vi "PSRR_PMIC.vi"() -> ()   [LabVIEW 2024]
panel:
  in  "MeasGraphs":enum32{"PSRR", "Hidden Controls"}(tab)
  out "Status":string
  out "PSRR vs Frequency":T1(graph)
  in  "Scope resource name":string
  in  "Fgen resource name":string
  in  "Load resource name":string
  in  "Source resource name":string caption="RESOURCE NAME"
  in  "MeasConfigurations":T2(tab)
  in  "Load sense":string="Remote" caption="LOAD SENSE"
  in  "Source sense":string="Remote" caption="SOURCE SENSE"
  in  "Nominal output voltage":dbl=3.3 caption="NOMINAL OUTPUT VOLTAGE" format="%#_6pV"
  in  "DUT setup time":dbl=1.0 caption="DUT SETUP TIME" format="%#_6ps"
  in  "Measurement settings":string="Measurement settings"
  in  "Source configuration":string="Source configuration"
  in  "Load configuration":string="Load configuration"
  in  "Load voltage limit":dbl=5.0 caption="VOLTAGE LIMIT" format="%#_6pV"
  in  "Load current level":dbl=0.05 caption="CURRENT LEVEL" format="%#_6pA"
  in  "Load resource name":refnum<k15> caption="RESOURCE NAME"
  in  "Source current limit":dbl=0.5 caption="CURRENT LIMIT" format="%#_6pA"
  in  "Source voltage level":dbl=20.0 caption="VOLTAGE LEVEL" format="%#_6pV"
  in  "Source resource name":refnum<k15> caption="RESOURCE NAME"
  in  "Scope vout range":dbl=0.05 caption="VOUT RANGE"
  in  "Scope input impedance":dbl=1000000.0 caption="INPUT IMPEDANCE" format="%#_6pOhm"
  in  "Scope number of cycles":i32=8 caption="NUMBER OF CYCLES"
  in  "Scope samples per cycle":i32=100000 caption="SAMPLES PER CYCLE"
  in  "Scope probe attenuation Vout":dbl=1.0 caption="VOUT PROBE ATTENUATION"
  in  "Scope output channel":string caption="OUTPUT CHANNEL NAME"
  in  "Scope maximum sample rate":dbl=100000000.0 caption="MAX SAMPLE RATE"
  in  "Scope minimum sample rate":dbl=100.0 caption="MIN SAMPLE RATE"
  in  "FGEN sweep type":string(combo)="Logarithmic" caption="SWEEP TYPE"
  in  "FGEN points or points per decade":i32=10 caption="PTS/PTS PER DECADE"
  in  "FGEN stop frequency":dbl=10000000.0 caption="STOP FREQUENCY" format="%#_6pHz"
  in  "FGEN start frequency":dbl=100.0 caption="START FREQUENCY" format="%#_6pHz"
  in  "FGEN load impedance":dbl=10000.0 caption="LOAD IMPEDANCE" format="%#_6pOhm"
  in  "Fgen configuration":string="Fgen configuration"
  in  "FGEN pk-pk amplitude":dbl=1.0 caption="PK-PK AMPLITUDE" format="%#_6pV"
  in  "FGEN channel name":string="0" caption="CHANNEL NAME"
  in  "FGEN resource name":refnum<k15> caption="RESOURCE NAME"
  in  "Scope probe attenuation Vin":dbl=1.0 caption="VIN PROBE ATTENUATION"
  in  "Scope configuration":string="Scope configuration"
  in  "Scope input channel":string caption="INPUT CHANNEL NAME"
  in  "Scope resource name":refnum<k15> caption="RESOURCE NAME"
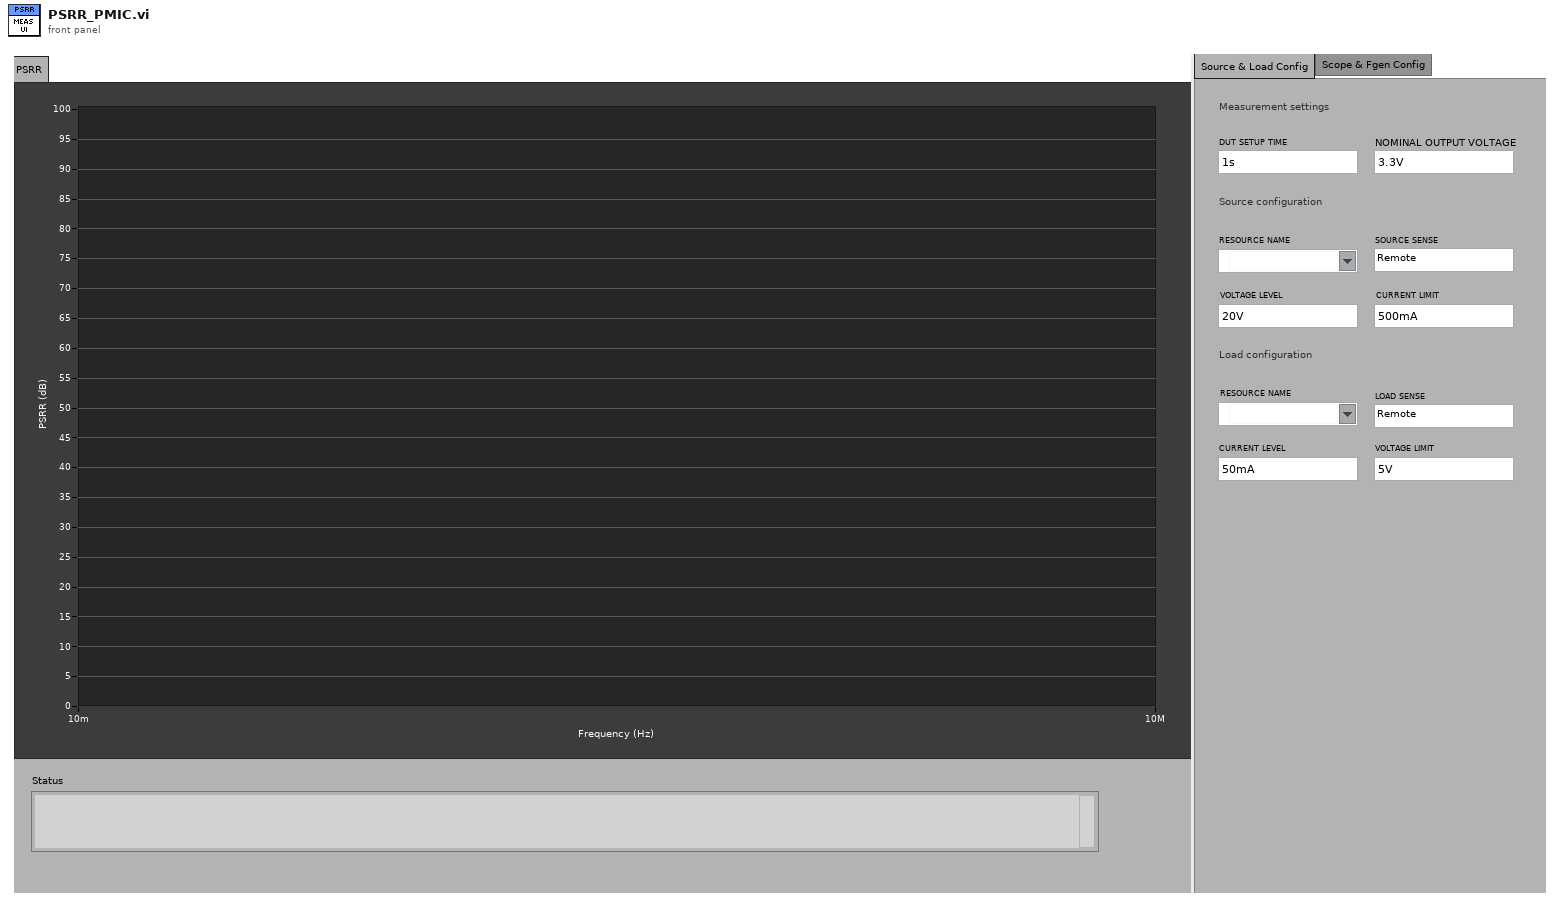
[diagram p1: front panel]
types:
  T1 = cluster{"Source voltages":dbl[], "Load voltages":dbl[]}
  T2 = enum32{"Source & Load Config", "Scope & Fgen Config"}
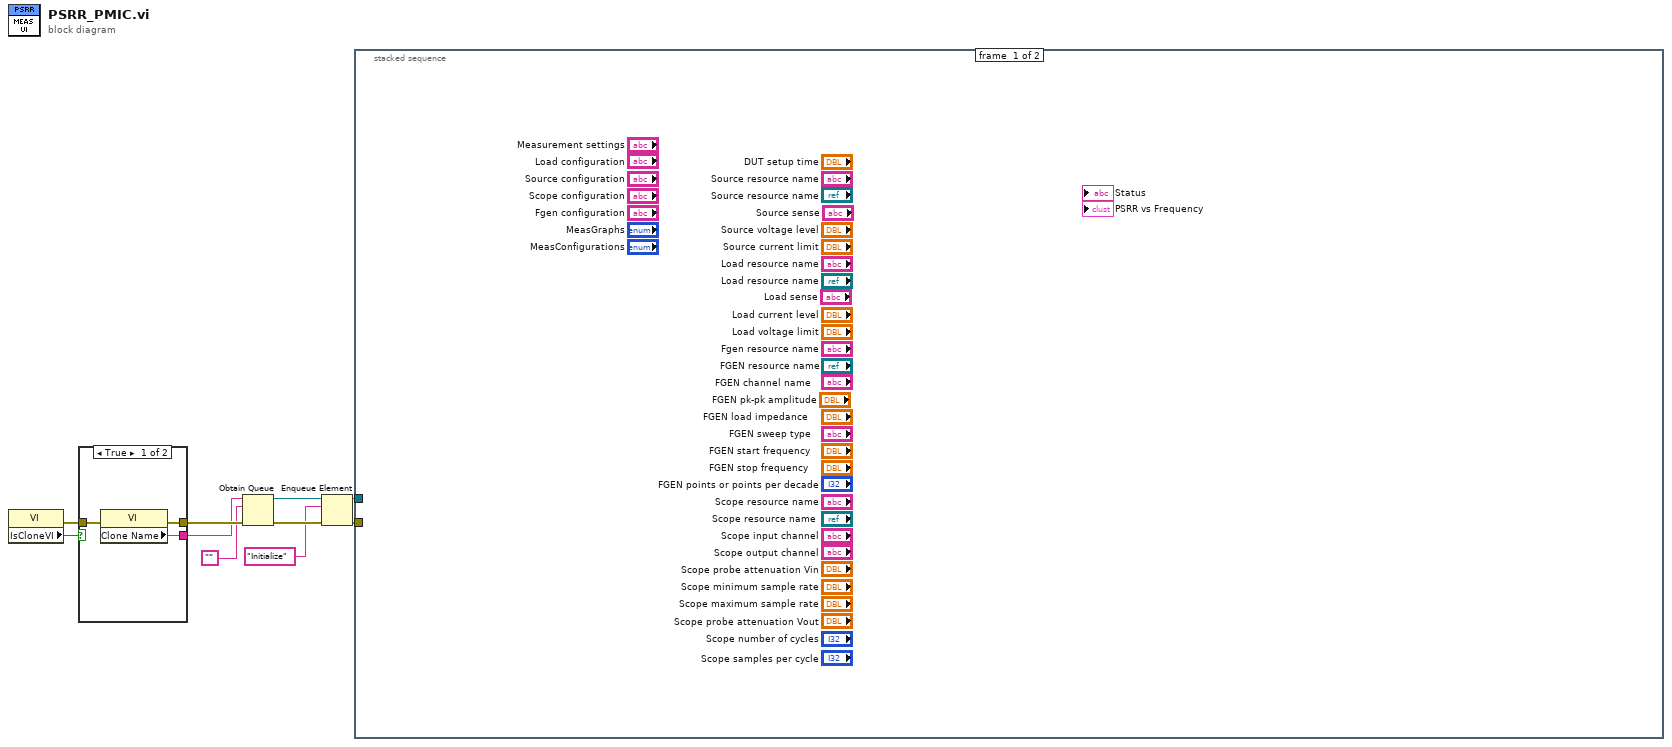
[diagram p0: block diagram]
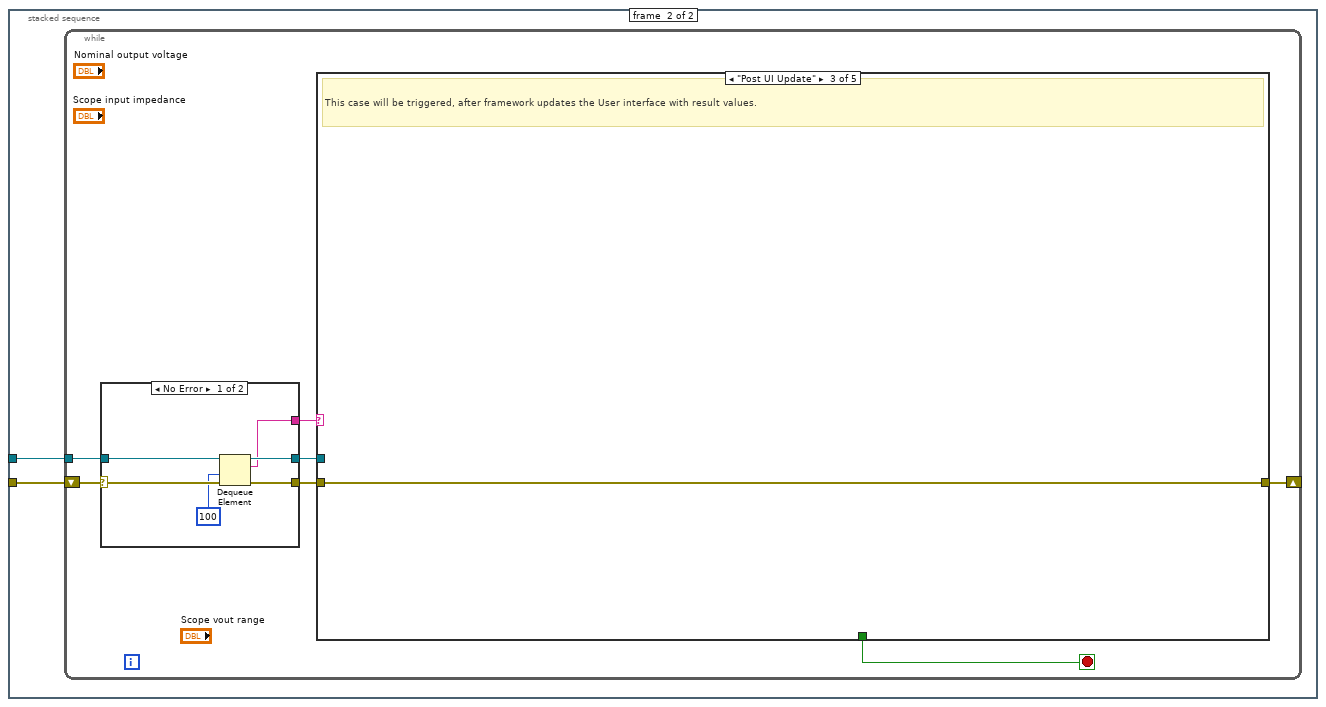
[diagram p2: hidden frame]
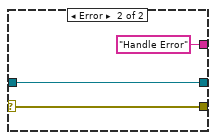
[diagram p3: hidden frame]
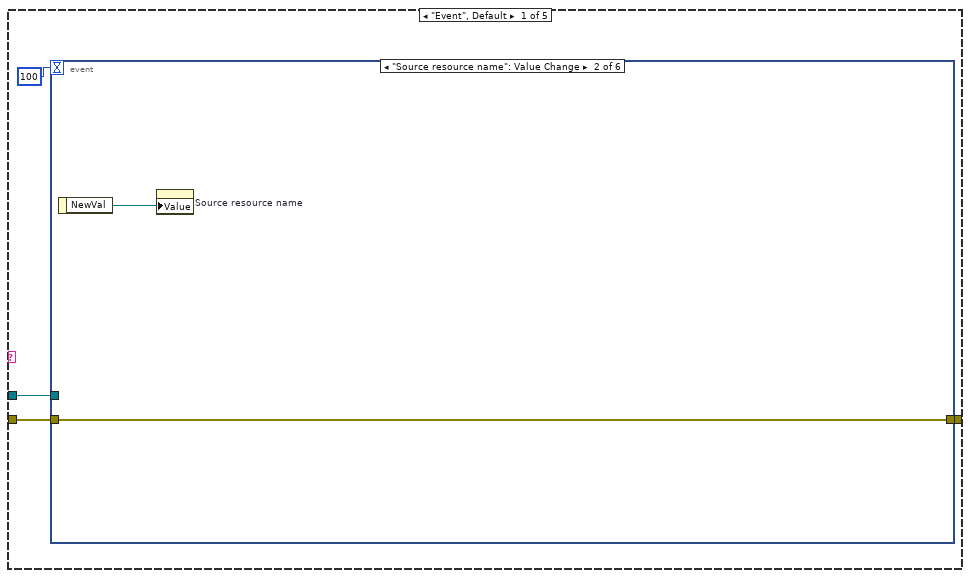
[diagram p4: hidden frame]
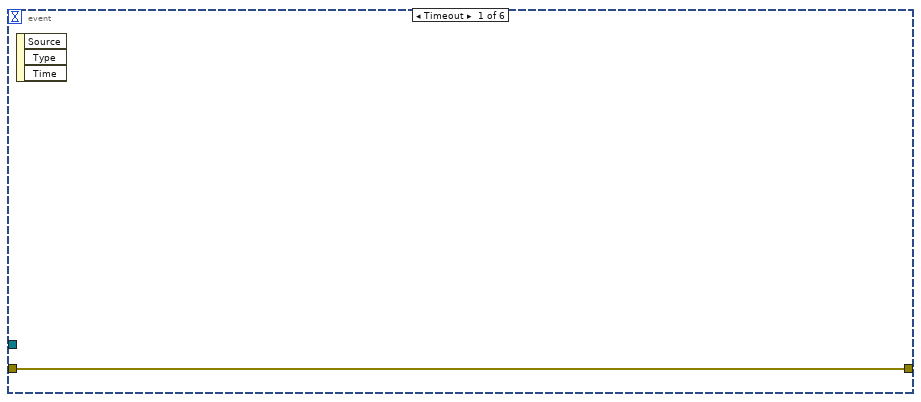
[diagram p5: hidden frame]
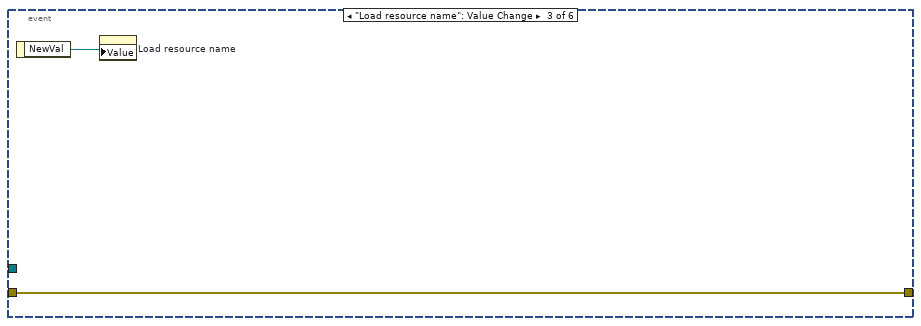
[diagram p6: hidden frame]
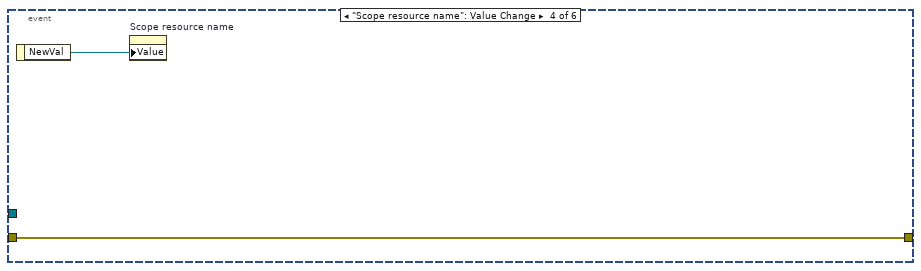
[diagram p7: hidden frame]
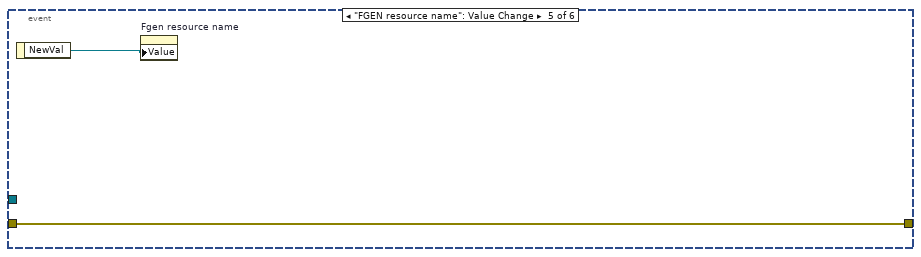
[diagram p8: hidden frame]
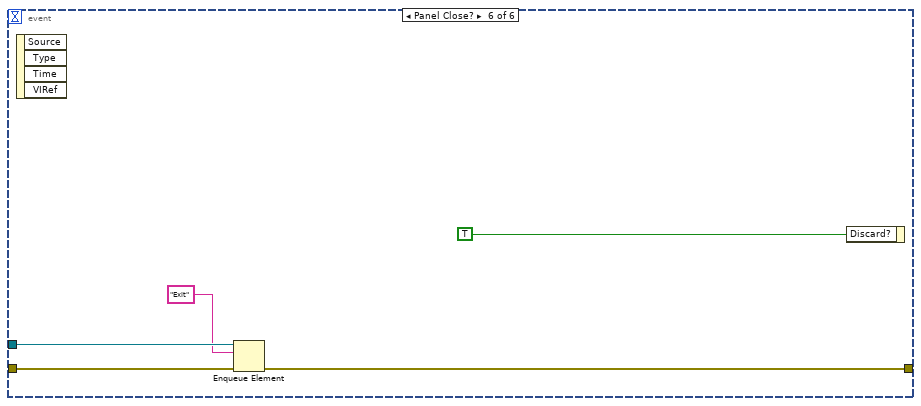
[diagram p9: hidden frame]
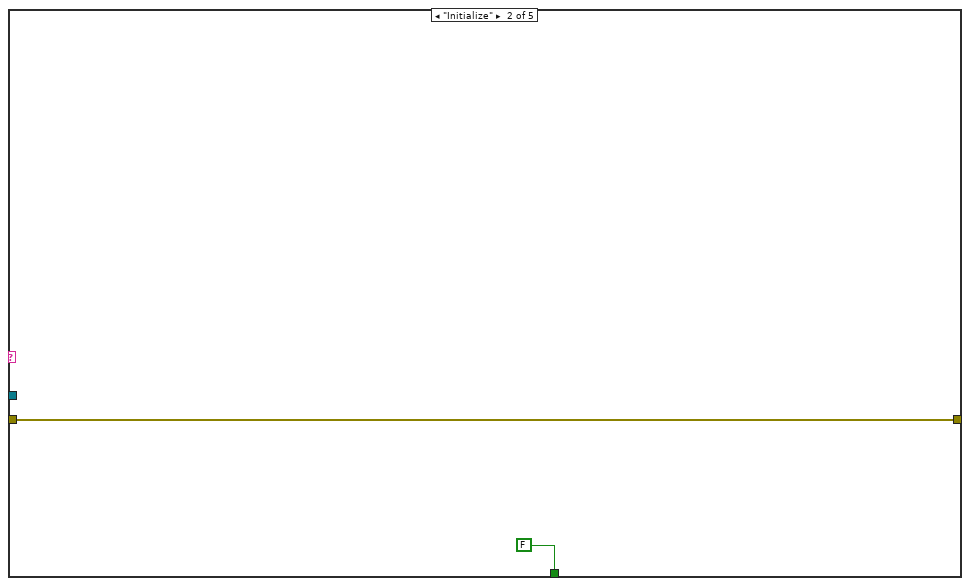
[diagram p10: hidden frame]
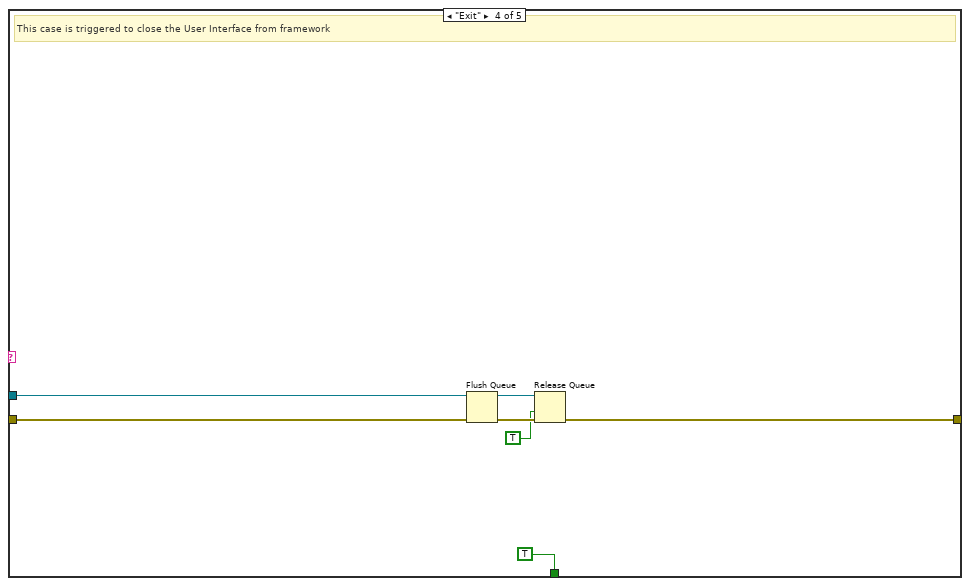
[diagram p11: hidden frame]
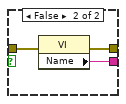
[diagram p13: hidden frame]
diagram:
  n1 = property class="VI"() -> (error out=w1:errorcluster, "IsCloneVI"=w2:bool)  [unwired: 2 in, 1 out]
  n2 = case shown="True" w2 {
    tunnel: [w13 w16] -> w10
    tunnel: [w12 w15] -> w9
    tunnel: w1 -> [w11 w14]
    frame True {
      n3 = property class="VI"(error in=w11) -> (error out=w13:errorcluster, "Clone Name"=w12:string)  [unwired: 1 in, 1 out]
    }
    frame False {
      n4 = property class="VI"(error in=w14) -> (error out=w16:errorcluster, "Name"=w15:string)  [unwired: 1 in, 1 out]
    }
  }
  n5 = Obtain Queue(name (unnamed)=w9, element data type="", error in (no error)=w10) -> (queue out=w6:refnum<queue>, error out=w8:errorcluster)  [unwired: 2 in, 1 out]
  n6 = Enqueue Element(queue=w6, element="Initialize", error in (no error)=w8) -> (queue out=w5:refnum<queue>, error out=w7:errorcluster)  [unwired: 1 in, 1 out]
  n7 = stacked-sequence {
    tunnel: w7 -> [_ w18]
    tunnel: w5 -> [_ w17]
    frame #0 {
    }
    frame #1 {
      n8 = while {
        shift-right: [w20] -> _
        shift-left: w18 -> [w25]
        tunnel: w17 -> [w23]
        stop <- w19 stop-if-true
        n9 = case shown="No Error" w25 {
          selector: w25 -> [w31 w34]
          tunnel: [w30 w34] -> w24
          tunnel: w23 -> [w29 w33]
          tunnel: [w28 w33] -> w22
          tunnel: [w27 "Handle Error"] -> w21
          frame No Error {
            n10 = Dequeue Element(queue=w29, timeout in ms (-1)=100, error in (no error)=w31) -> (queue out=w28:refnum<queue>, element=w27:string, error out=w30:errorcluster)  [unwired: 1 out]
          }
          frame Error {
          }
        }
        n11 = case shown="\"Post UI Update\"" w21 {
          tunnel: w24 -> [w37 w54 w55 w62 w63]
          tunnel: w22 -> [w35 _ _ w60 _]
          tunnel: [w38 w54 w55 w57 w63] -> w20
          tunnel: [_ FALSE _ TRUE _] -> w19
          frame "Event", Default {
            n12 = event shown="[1] \"Source resource name\": Value Change" {
              selector: _ -> [_ _ _ _ _ _]
              dyn-events: _ -> [_ _ _ _ _ _]
              timeout: 100 -> [_ _ _ _ _ _]
              tunnel: [w39 w40 w42 w44 w46 w50] -> w38
              tunnel: w37 -> [w39 w40 w42 w44 w46 w51]
              tunnel: w35 -> [_ _ _ _ _ w49]
              event Timeout {
                n13 = event-data() -> ()  [unwired: 1 in, 3 out]
              }
              event "Source resource name": Value Change {
                n14 = event-data() -> ("NewVal"=w41:refnum<k15>)  [unwired: 1 in]
                n15 = property on="Source resource name" class="Str"("Value"=w41) -> ()  [unwired: 2 in, 2 out]
              }
              event "Load resource name": Value Change {
                n16 = event-data() -> ("NewVal"=w43:refnum<k15>)  [unwired: 1 in]
                n17 = property on="Load resource name" class="Str"("Value"=w43) -> ()  [unwired: 2 in, 2 out]
              }
              event "Scope resource name": Value Change {
                n18 = event-data() -> ("NewVal"=w45:refnum<k15>)  [unwired: 1 in]
                n19 = property on="Scope resource name" class="Str"("Value"=w45) -> ()  [unwired: 2 in, 2 out]
              }
              event "FGEN resource name": Value Change {
                n20 = event-data() -> ("NewVal"=w47:refnum<k15>)  [unwired: 1 in]
                n21 = property on="Fgen resource name" class="Str"("Value"=w47) -> ()  [unwired: 2 in, 2 out]
              }
              event Panel Close? {
                n22 = event-data() -> ()  [unwired: 1 in, 4 out]
                n23 = Enqueue Element(queue=w49, element="Exit", error in (no error)=w51) -> (error out=w50:errorcluster)  [unwired: 1 in, 2 out]
                n24 = event-data("Discard?"=TRUE) -> ()  [unwired: 1 in, 1 out]
              }
            }
          }
          frame "Initialize" {
          }
          frame "Post UI Update" {
            # "This case will be triggered, after framework updates the User interface with result values."
          }
          frame "Exit" {
            # "This case is triggered to close the User Interface from framework"
            n25 = Flush Queue(queue=w60, error in (no error)=w62) -> (queue out=w59:refnum<queue>, error out=w58:errorcluster)  [unwired: 1 out]
            n26 = Release Queue(queue=w59, force destroy? (F)=TRUE, error in (no error)=w58) -> (error out=w57:errorcluster)  [unwired: 2 out]
          }
          frame "Handle Error" {
          }
        }
      }
    }
  }
